vi "SOUR_POW_CENT.vi"(0 "VISA IN":refnum<visa-resource-name>, 1 "Center Power":i32, 5 "error in":errorcluster, 7 "Channel":i32) -> (14 "VISA Out":refnum<visa-resource-name>, 19 "error out":errorcluster)   [LabVIEW 2018, in "PNA-X.lvlib"]
doc: "SOURce<cnum>:POWer:CENTer <num> \n1827\n\n(Read-Write) Sets the power sweep center power. Must also set: \nSENS:SWE:TYPE POWer and SOURce:POWer:SPAN <num>. \nParameters \n<cnum> Any existing channel number. If unspecified, value is set to 1 \n<num> Center power. Actual achievable leveled power depends on frequency. \nExamples SOUR:POW:CENT -15 \nsource2:power:center -7 \nQuery Syntax SOURce<cnum>:POWer:CENTer? \nReturn Type Numeric \nDefault 0 dBm"
uses:
  PNA-X.lvlib
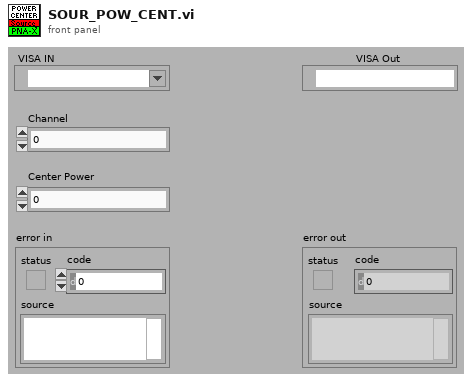
[diagram p1: front panel]
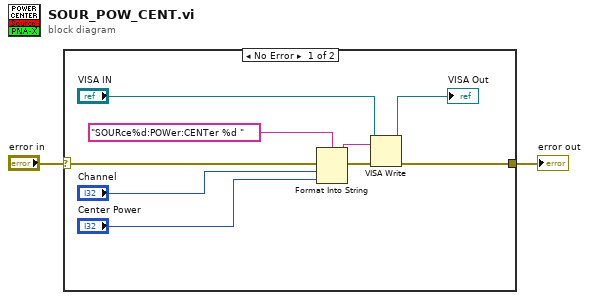
[diagram p0: block diagram]
diagram:
  n1 = case shown="No Error" "error in" {
    selector: "error in" -> [w11 w12]
    tunnel: [w6 w12] -> w1
    frame No Error {
      n2 = Format Into String(format string="SOURce%d:POWer:CENTer %d " ("Cmdline"), error in=w11, "Channel", "Center Power") -> (resulting string=w9:string, error out=w10:errorcluster)  [unwired: 1 in]
      n3 = VISA Write(VISA resource name="VISA IN", write buffer=w9, error in (no error)=w10) -> (VISA resource name out=→"VISA Out":refnum<visa-resource-name>, error out=w6:errorcluster)  [unwired: 1 out]
    }
    frame Error {
    }
  }
  "error out" <- w1
